vi "Set Anonymous User.vi"(8 "error in (no error)":errorcluster, 11 "Processing in":refnum<class "Processing.lvclass">) -> (0 "error out":errorcluster, 3 "Processing out":refnum<class "Processing.lvclass">)   [LabVIEW 2020, in "HTTP Server.lvlib" / "Processing.lvclass"]
uses:
  Processing.lvclass
  Security/Security.lvclass
  Values/Values.lvclass
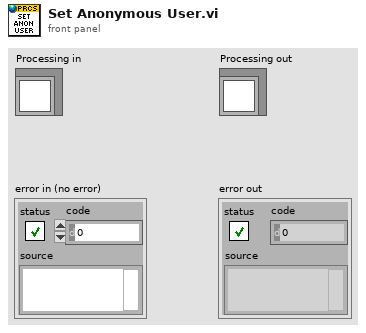
[diagram p1: front panel]
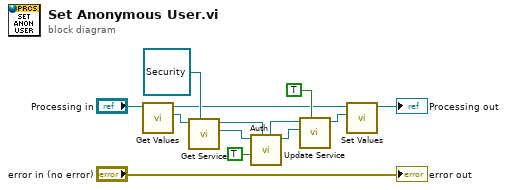
[diagram p0: block diagram]
diagram:
  n1 = call "Get Values.vi"("Processing in"="Processing in") -> ("Values"=w12:refnum<class "Values.lvclass">, "Processing out"=w7:refnum<class "Processing.lvclass">)  [unwired: 9 in]
  n2 = call "Get Service.vi"("Service Type"=refnum<class "Security.lvclass"> refnum ("Security in"), "Values in"=w12) -> ("Service"=w10:refnum<class "Security.lvclass">, "Values out"=w5:refnum<class "Values.lvclass">)  [unwired: 7 in, 1 out]
  n3 = call "Auth.vi"("Values In"=w5, "Anonymous (F)"=TRUE, "Security in"=w10) -> ("Security out"=w9:refnum<class "Security.lvclass">, "Values"=w4:refnum<class "Values.lvclass">)  [unwired: 6 in, 1 out]
  n4 = call "Update Service.vi"("Overwrite? (F)"=TRUE, "Service"=w9, "Values in"=w4) -> ("Values out"=w6:refnum<class "Values.lvclass">)  [unwired: 7 in, 1 out]
  n5 = call "Set Values.vi"("Values"=w6, "Processing in"=w7) -> ("Processing out"=→"Processing out":refnum<class "Processing.lvclass">)  [unwired: 9 in]
  "error out" <- "error in (no error)"
